vi "0816039.vi"() -> ()   [LabVIEW 2021]
panel:
  in  "stop":bool
  out "1":T1={"[0]"=TRUE, "[1]"=TRUE, "[2]"=TRUE, "[3]"=FALSE, "[4]"=FALSE, "[5]"=TRUE, "[6]"=TRUE}
  in  "OK Button":bool
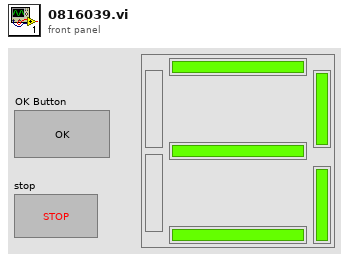
[diagram p1: front panel]
types:
  T1 = cluster{"[0]":bool, "[1]":bool, "[2]":bool, "[3]":bool, "[4]":bool, "[5]":bool, "[6]":bool}
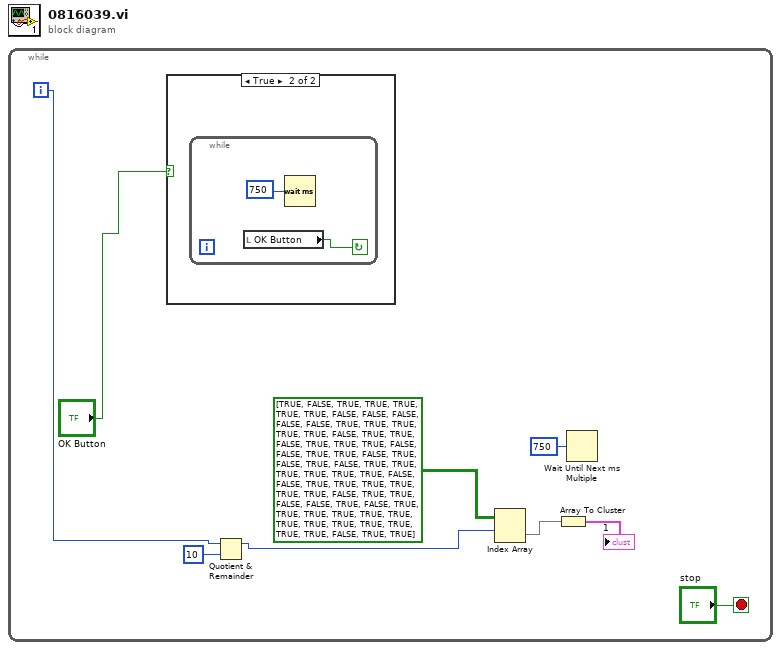
[diagram p0: block diagram]
diagram:
  n1 = while {
    i -> [w2]
    stop <- "stop" stop-if-true
    n2 = case shown="True" "OK Button" {
      frame False {
      }
      frame True {
        n3 = while {
          stop <- w10 continue-if-true
          n4 = local read "OK Button"() -> (w10:bool)
          n5 = Wait (ms)(milliseconds to wait=u32 750) -> ()  [unwired: 1 out]
        }
      }
    }
    n6 = Quotient & Remainder(x=w2, y=10) -> (x-y*floor(x/y)=w3:i32)  [unwired: 1 out]
    n7 = Index Array "Index Array"(array=bool[][] [[TRUE, FALSE, TRUE, TRUE, TRUE, TRUE, TRUE], [FALSE, FALSE, FALSE, FALSE, FALSE, TRUE, TRUE], [TRUE, TRUE, TRUE, FALSE, TRUE, TRUE, FALSE], [TRUE, TRUE, TRUE, FALSE, FALSE, TRUE, TRUE], [FALSE, TRUE, FALSE, TRUE, FALSE, TRUE, TRUE], [TRUE, TRUE, TRUE, TRUE, FALSE, FALSE, TRUE], [TRUE, TRUE, TRUE, TRUE, TRUE, FALSE, TRUE], [TRUE, FALSE, FALSE, TRUE, FALSE, TRUE, TRUE], [TRUE, TRUE, TRUE, TRUE, TRUE, TRUE, TRUE], [TRUE, TRUE, TRUE, TRUE, FALSE, TRUE, TRUE]], index (row)=w3) -> (element=w5:bool[])  [unwired: 1 in]
    n8 = Array To Cluster(array=w5) -> (cluster=→"1":T1)
    n9 = Wait Until Next ms Multiple(millisecond multiple=u32 750) -> ()  [unwired: 1 out]
  }
